vi "Autonomous Independent.vi"() -> ()   [LabVIEW 2016]
doc: "This VI is called when autonomous begins, and will automatically be terminated when autonomous ends. You can carry out timed or sensor driven robot movement independently without needing to return to the caller."
uses:
  <vilib>/Rock Robotics/WPI/Solenoid/WPI_SolenoidValue.ctl
  <vilib>/Rock Robotics/WPI/Utilities/WPI_GetSetVariantRefNum.vi
  <vilib>/Rock Robotics/Network Tables/NT Read String.vi
  <vilib>/Rock Robotics/Network Tables/NT Read Boolean.vi
  <vilib>/Rock Robotics/WPI/Solenoid/WPI_SolenoidSetEnum.vi
  <vilib>/Rock Robotics/WPI/RobotDrive/WPI_RobotDriveArcadeDrive_Standard(NoSaturation).vi
  <vilib>/Rock Robotics/Network Tables/NT Write Numeric Array.vi
  <vilib>/Rock Robotics/Network Tables/NT Write Number.vi
  Google Drive/HowdyBots-Share/BotStuff/2017_SteamWorks/Code/BotCode/Active/Robot Global Data.vi
  <vilib>/Rock Robotics/WPI/Counter/WPI_CounterDigitalInputToDigitalSource.vi
  <vilib>/Rock Robotics/SystemInterfaces/DIO/FPGA_DIOChannel.ctl
panel:
  out "Hook Center Cons":dbl
  out "gyro":dbl
  out "sonar distance (inches)":dbl
  out "Encoder Loop":dbl
  out "Encoder Loop":string
  out "Current Movement, for debugging 2":T1 {"Y Joystick Value" scale=1.0..-1.0; "X Joystick Value" scale=-1.0..1.0}
  in  "Array of robot movements 2":T2(array[cluster])=[{"X Joystick Value"=0.39393939393939403, "Y Joystick Value"=0.0, "Delay (sec)"=1.0, "Movement Name"="turn"}, {"X Joystick Value"=-0.3737373737373737, "Y Joystick Value"=0.0, "Delay (sec)"=1.0, "Movement Name"="turn back"}] {"Y Joystick Value" scale=1.0..-1.0; "X Joystick Value" scale=-1.0..1.0}
  # "Sensor Readings\nConstanly updated in\nwhile loopes"
  # "Be sure to right-click and choose Data Operations>>Make Current Value default if you want to save the array values with the VI"
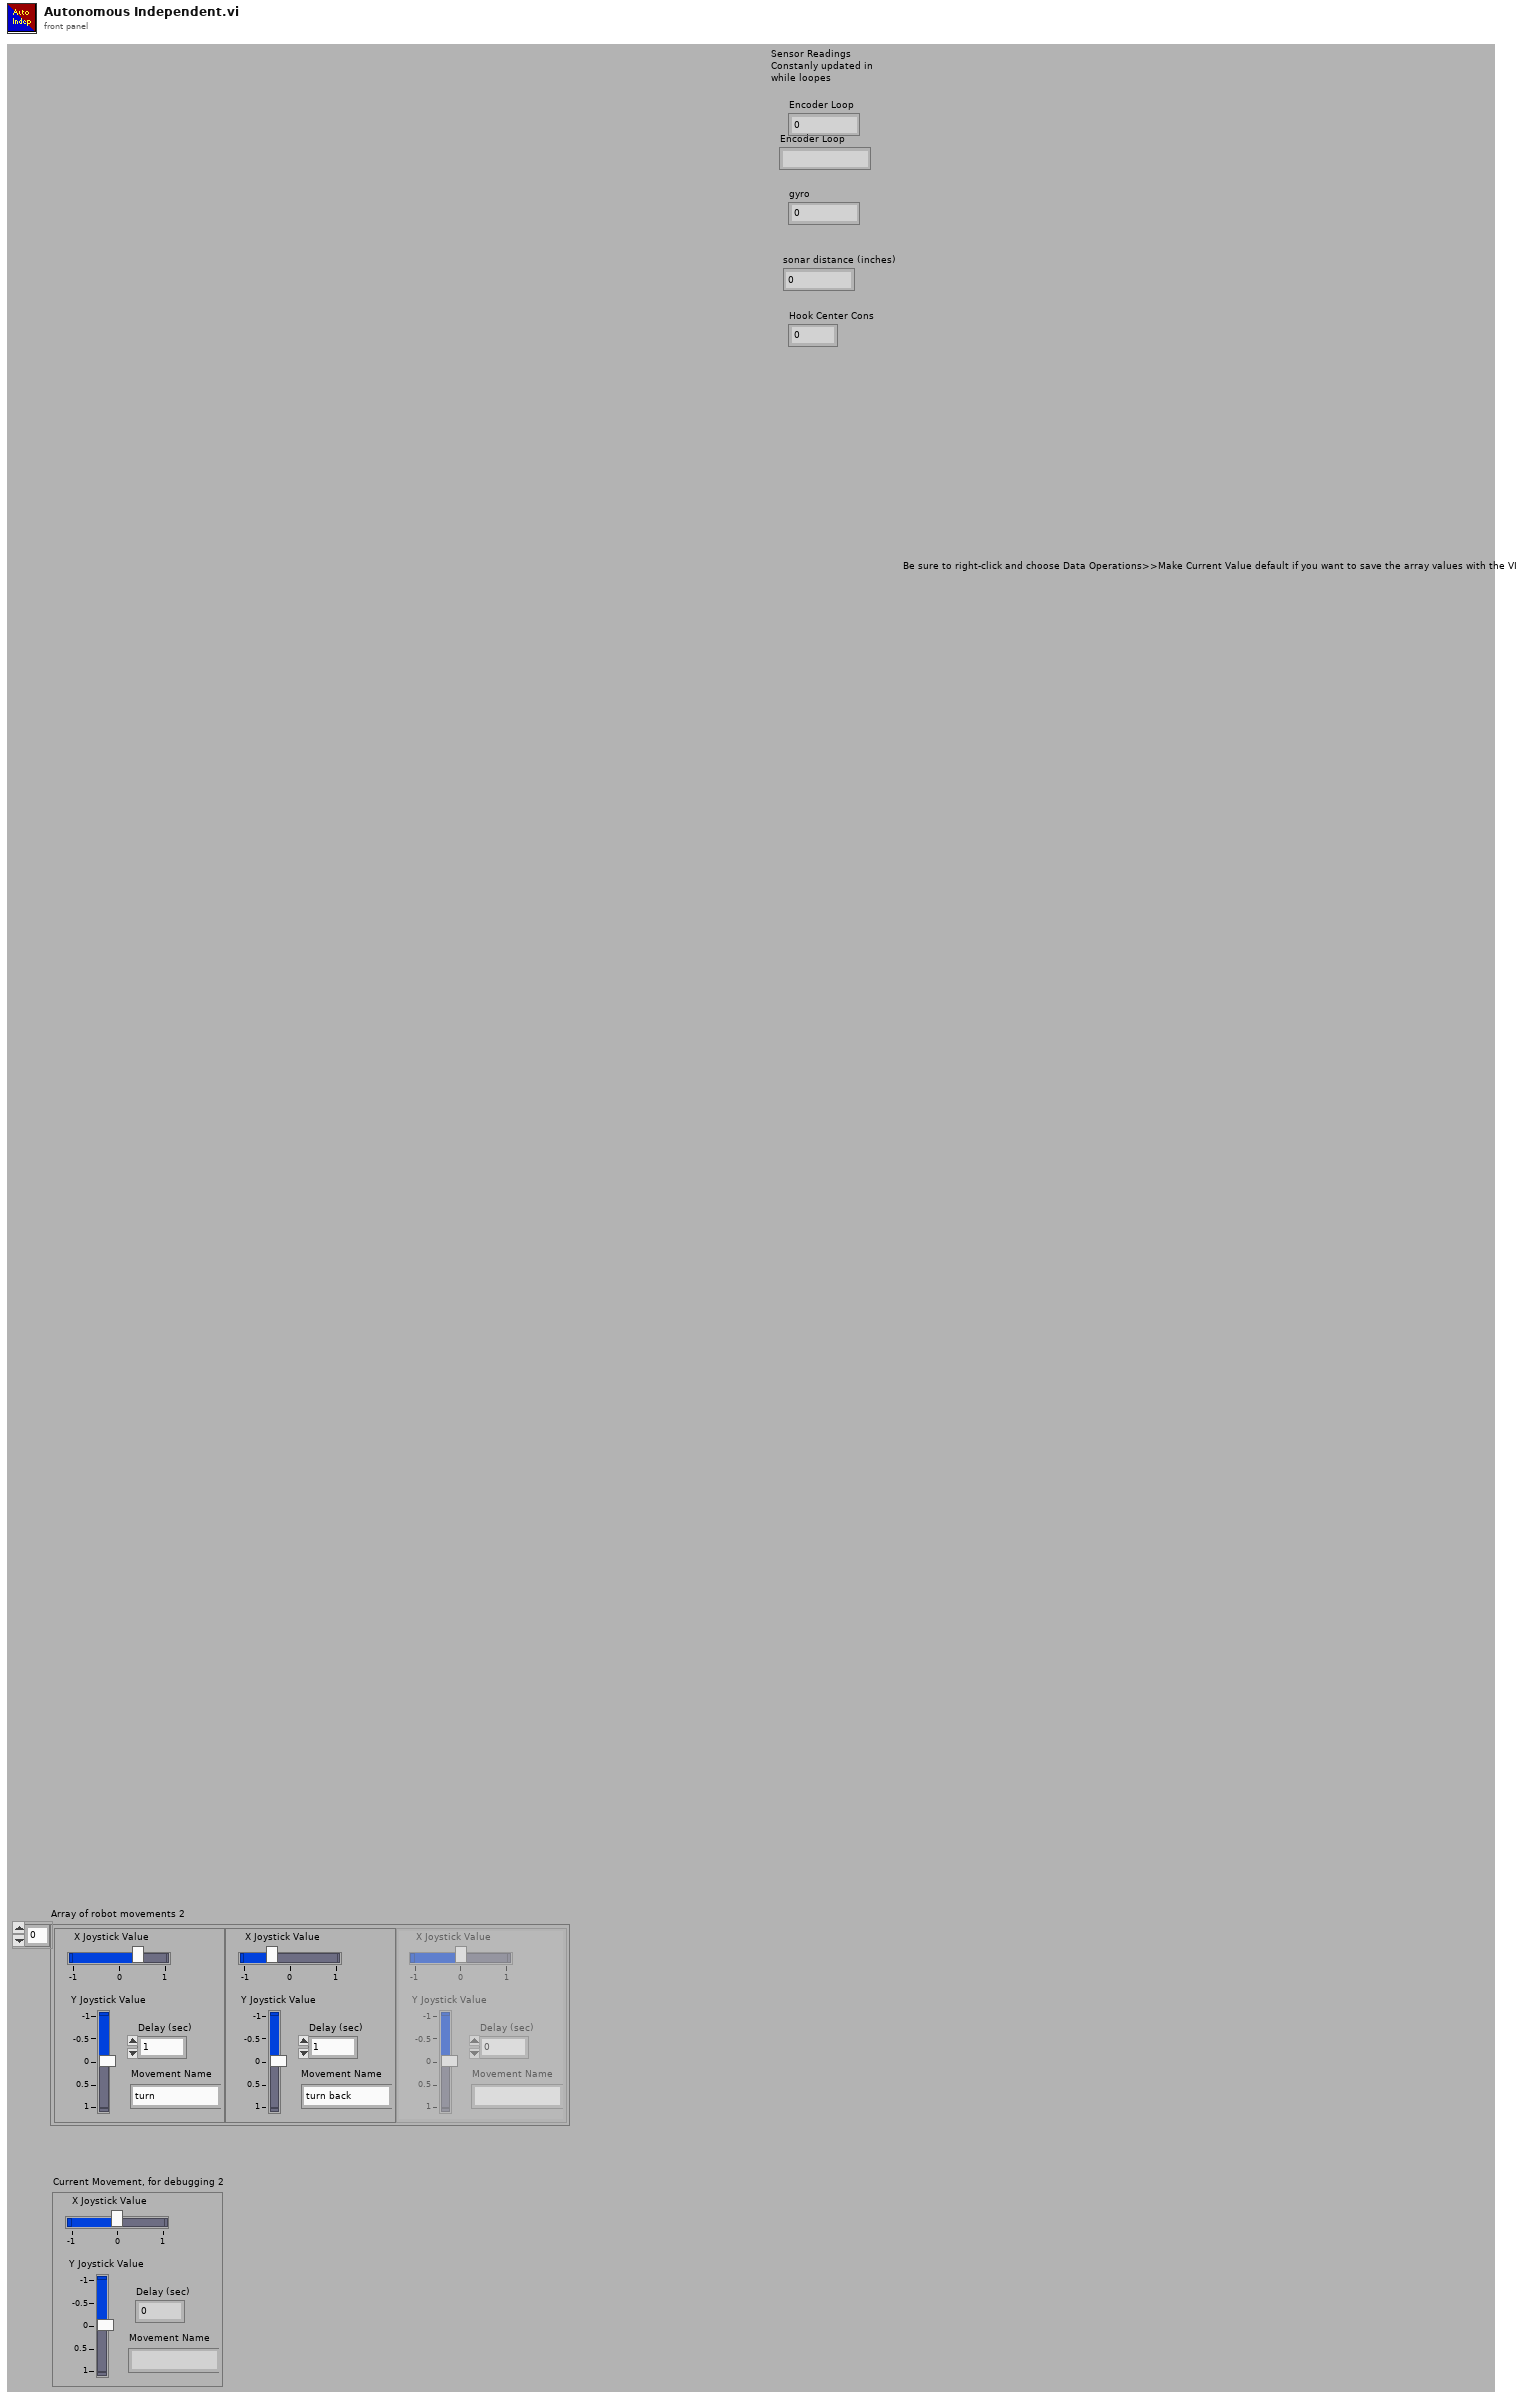
[diagram p1: front panel]
types:
  T1 = cluster{"X Joystick Value":dbl, "Y Joystick Value":dbl, "Delay (sec)":dbl, "Movement Name":string}
  T2 = cluster{"X Joystick Value":dbl, "Y Joystick Value":dbl, "Delay (sec)":dbl, "Movement Name":string}[]
  T3 = typedef "FPGA_DIOChannel.ctl" = enum8{"DIO 0", "DIO 1", "DIO 2", "DIO 3", "DIO 4", "DIO 5", "DIO 6", "DIO 7", "DIO 8", "DIO 9", "DIO MXP 0", "DIO MXP 1", "DIO MXP 2", "DIO MXP 3", "DIO MXP 4", "DIO MXP 5", "DIO MXP 6", "DIO MXP 7", "DIO MXP 8", "DIO MXP 9", "DIO MXP 10", "DIO MXP 11", "DIO MXP 12", "DIO MXP 13", "DIO MXP 14", "DIO MXP 15", "SPI Port CS1", "SPI Port CS2", "SPI Port CS3", "SPI Port MISO", "SPI Port MOSI", "Invalid"}
  T4 = typedef "WPI_DigitalInputDevRef.ctl" = cluster{"DevStatus":errorcluster, "DIO Channel":T3}
  T5 = typedef "FPGA_CounterEncoderSourceConvertionLVSourceType.ctl" = cluster{"DevStatus":errorcluster, "AnalogTriggerMode?":bool, "DigitalMode":cluster{"DIO Channel":T6}, "AnalogTriggerMode":cluster{"AnalogTriggerIndex":T7, "OutputType":T8}}
  T6 = typedef "FPGA_DIODigitalSourceChannel.ctl" = enum8{"DIO 0", "DIO 1", "DIO 2", "DIO 3", "DIO 4", "DIO 5", "DIO 6", "DIO 7", "DIO 8", "DIO 9", "DIO MXP 0", "DIO MXP 1", "DIO MXP 2", "DIO MXP 3", "DIO MXP 4", "DIO MXP 5", "DIO MXP 6", "DIO MXP 7", "DIO MXP 8", "DIO MXP 9", "DIO MXP 10", "DIO MXP 11", "DIO MXP 12", "DIO MXP 13", "DIO MXP 14", "DIO MXP 15", "Disabled"}
  T7 = typedef "FPGA_AnalogTriggerIndex.ctl" = enum8{"Trig 0", "Trig 1", "Trig 2", "Trig 3", "Trig 4", "Trig 5", "Trig 6", "Trig 7", "Invalid"}
  T8 = typedef "FPGA_AnalogTriggerOutType.ctl" = enum16{"InWindow", "TriggerState", "Rising", "Falling"}
  T9 = typedef "WPI_EncoderDevRef.ctl" = cluster{"DevStatus":errorcluster, "EncoderIndex":T10, "CounterIndex":T11, "DistancePerCount":dbl, "Decoding Type":T12}
  T10 = typedef "FPGA_EncoderIdx.ctl" = enum8{"Enc 0", "Enc 1", "Enc 2", "Enc 3", "Enc 4", "Enc 5", "Enc 6", "Enc 7", "Invalid"}
  T11 = typedef "FPGA_CounterCtrSystemIndex.ctl" = enum8{"Ctr 0", "Ctr 1", "Ctr 2", "Ctr 3", "Ctr 4", "Ctr 5", "Ctr 6", "Ctr 7", "Invalid"}
  T12 = typedef "WPI_EncoderType.ctl" = enum16{"1x", "2x", "4x"}
  T13 = typedef "WPI_JoystickDevRef.ctl" = cluster{"Device":T14}
  T14 = typedef "WPI_JoystickDeviceEnum.ctl" = enum16{"USB 0", "USB 1", "USB 2", "USB 3", "USB 4", "USB 5"}
  T15 = typedef "WPI_SolenoidValue.ctl" = enum16{"Off", "On", "Forward", "Reverse"}
  T16 = typedef "WPI_SolenoidDevRef.ctl" = cluster{"DevStatus":errorcluster, "Pneumatics Control Module":u8, "Forward Solenoid Channel":T17, "Reverse Solenoid Channel":T17}
  T17 = typedef "WPI_SolenoidChannel.ctl" = enum8{"Solenoid 0", "Solenoid 1", "Solenoid 2", "Solenoid 3", "Solenoid 4", "Solenoid 5", "Solenoid 6", "Solenoid 7", "Invalid"}
  T18 = typedef "WPI_RobotDriveDevRef.ctl" = cluster{"DevStatus":errorcluster, "Motors[]":T19[], "Square Inputs":bool, "Max Output":dbl}
  T19 = typedef "WPI_MotorControlDeviceRef.ctl" = cluster{"DeviceStatus":errorcluster, "Type":T20, "PWM":cluster{"PWM Channel":T21, "DeadBand":T22}, "CAN":cluster{"Device Number":u8, "SetOutput VI Ref":variant, "GetOutput VI Ref":variant, "Enable VI Ref":variant, "Disable VI Ref":variant, "Data":variant}, "Invert":bool}
  T20 = typedef "WPI_MotorControlType.ctl" = enum16{"PWM", "CAN"}
  T21 = typedef "FPGA_DIOPWMChannel.ctl" = enum8{"PWM 0", "PWM 1", "PWM 2", "PWM 3", "PWM 4", "PWM 5", "PWM 6", "PWM 7", "PWM 8", "PWM 9", "PWM MXP 0", "PWM MXP 1", "PWM MXP 2", "PWM MXP 3", "PWM MXP 4", "PWM MXP 5", "PWM MXP 6", "PWM MXP 7", "PWM MXP 8", "PWM MXP 9", "Invalid"}
  T22 = typedef "WPI_PWMDeadband.ctl" = cluster{"Name":string, "maxPositivePwm":i32, "minPositivePwm":i32, "centerPwm":i32, "maxNegativePwm":i32, "minNegativePwm":i32, "angularRange":u16}
  T23 = typedef "WPI_DriverStationPositionInfo.ctl" = enum16{"1", "2", "3"}
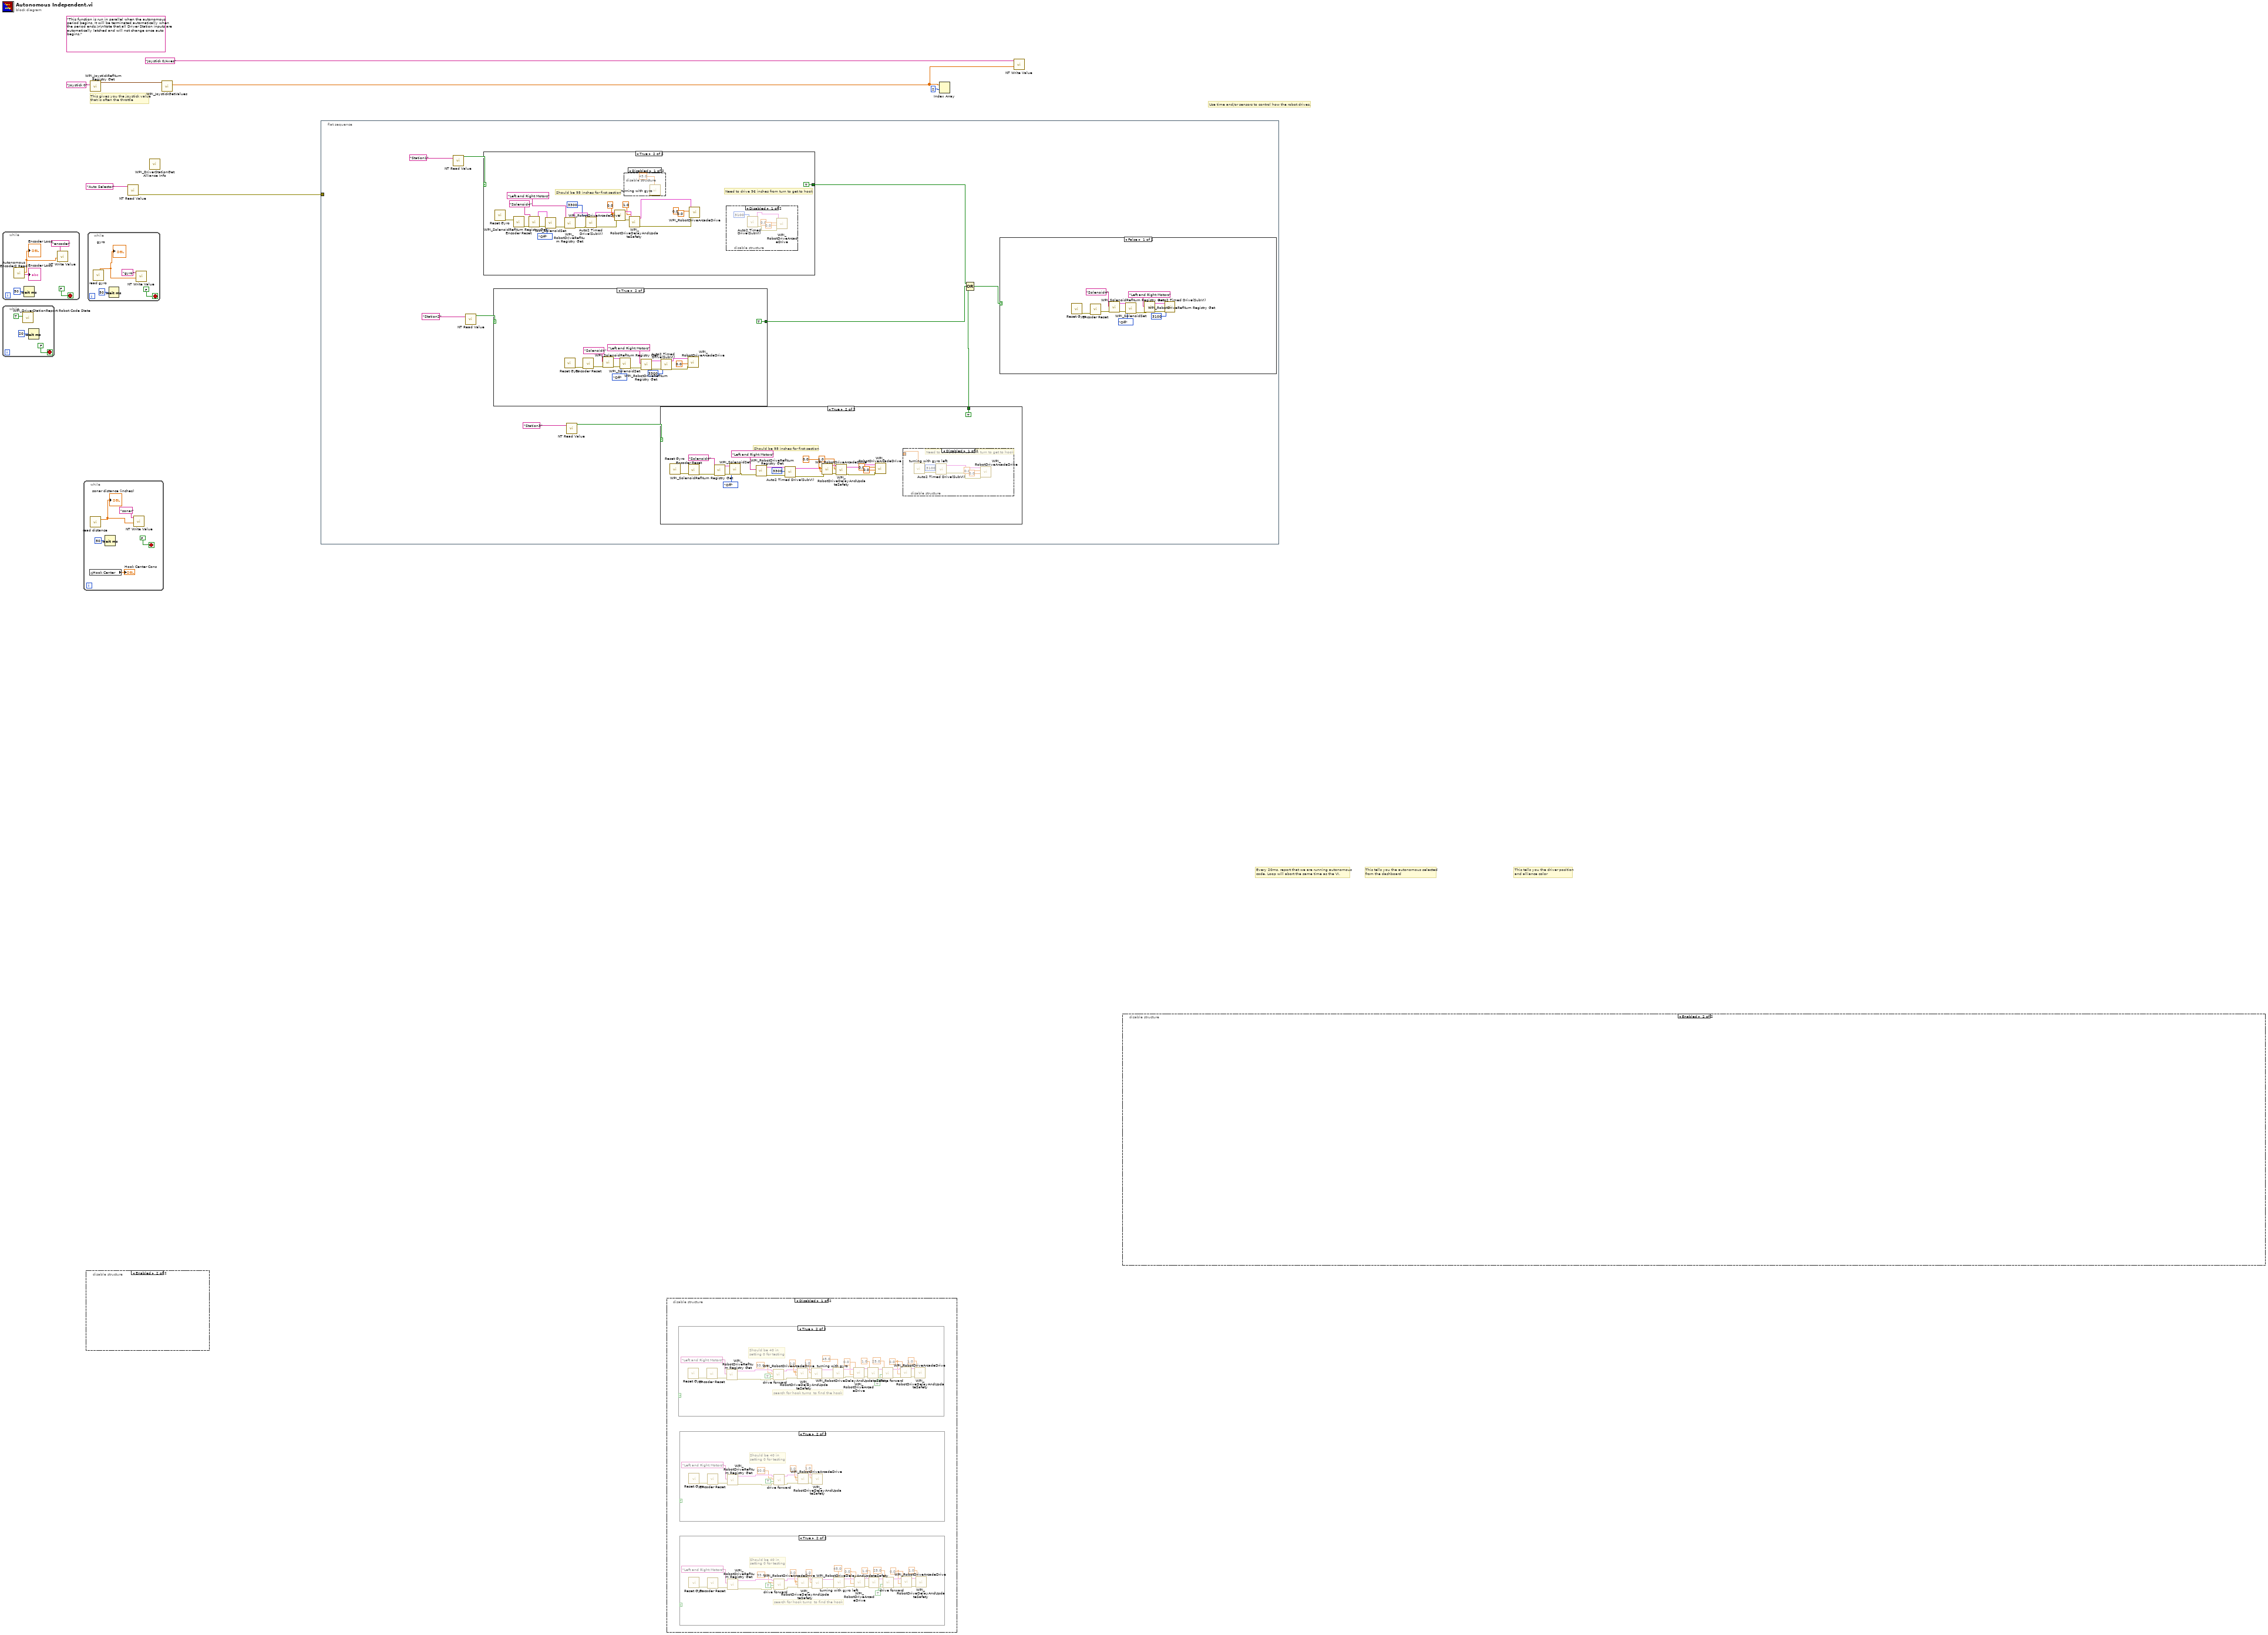
[diagram p0: block diagram]
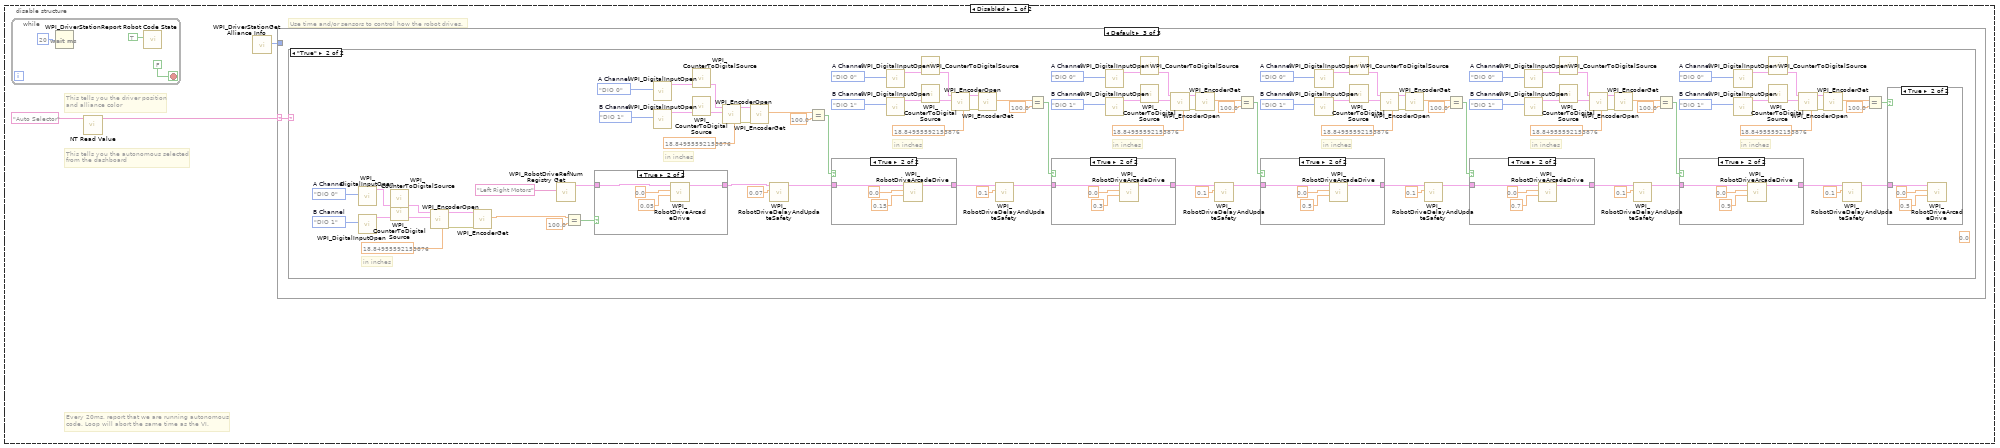
[diagram p13: hidden frame]
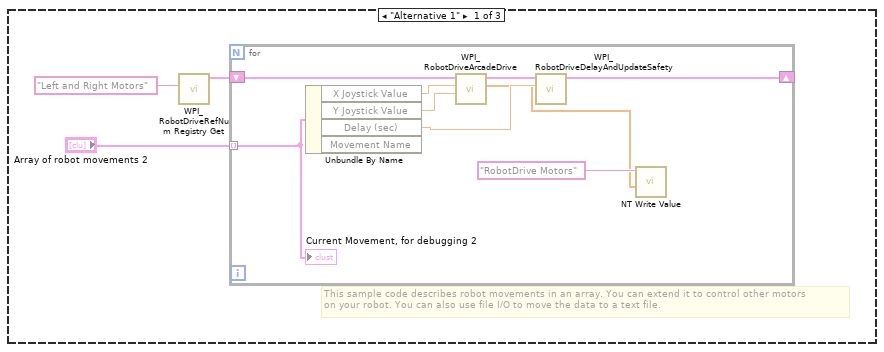
[diagram p14: hidden frame]
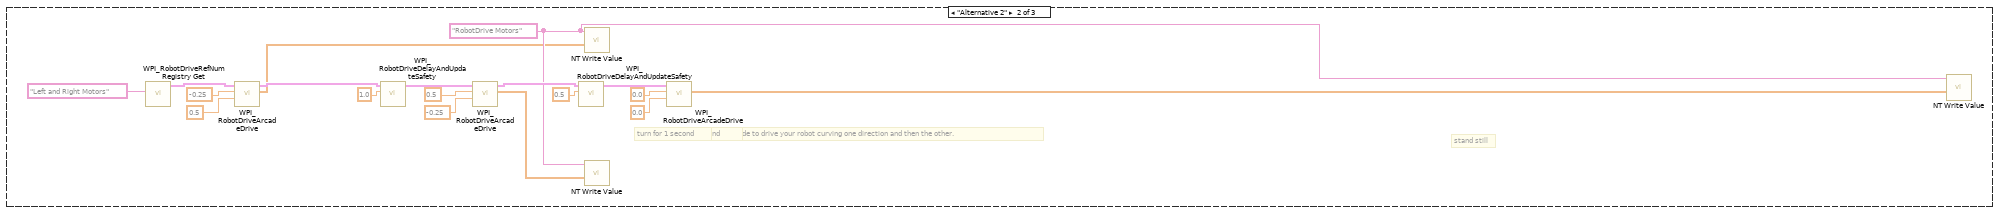
[diagram p15: hidden frame]
diagram:
  (unwired) "This function is run in parallel when the autonomous period begins. It will be terminated automatically when the period ends.\n\nNote that all Driver Station inputs are automatically latched and will not change once auto begins."
  # "This tells you the autonomous selected\nfrom the dashboard"
  # "Every 20ms, report that we are running autonomous\ncode. Loop will abort the same time as the VI."
  # "This gives you the joystick value\nthat is often the throttle"
  # "Use time and/or sensors to control how the robot drives."
  # "This tells you the driver position\nand alliance color"
  n1 = while {
    stop <- FALSE stop-if-true
    n2 = call "Autonomous Encoder2 Read.vi"() -> ("Encoder Direction"=→"Encoder Loop":string, "Encoder Distance"=w9:dbl)  [unwired: 9 in, 1 out]
    "Encoder Loop" <- w9
    n3 = Wait (ms)(milliseconds to wait=u32 50) -> ()  [unwired: 1 out]
    n4 = call-poly <vilib>:"NT Write Value.vi"("Numeric"=w9, "Name"="encoder") -> ()  [unwired: 9 in, 1 out]
  }
  n5 = while {
    stop <- FALSE stop-if-true
    n6 = call <vilib>:"WPI_DriverStationReport Robot Code State.vi"("Autonomous"=TRUE) -> ()  [unwired: 10 in, 1 out]
    n7 = Wait (ms)(milliseconds to wait=u32 20) -> ()  [unwired: 1 out]
  }
  n8 = while {
    stop <- FALSE stop-if-true
    n9 = global read "Robot Global Data.vi" "Hook Center"() -> (→"Hook Center Cons":dbl)
    n10 = call "read distance.vi"() -> ("Distance 2"=w18:dbl)  [unwired: 10 in, 1 out]
    "sonar distance (inches)" <- w18
    n11 = Wait (ms)(milliseconds to wait=u32 50) -> ()  [unwired: 1 out]
    n12 = call-poly <vilib>:"NT Write Value.vi"("Numeric"=w18, "Name"="sonar") -> ()  [unwired: 9 in, 1 out]
  }
  n13 = disable-structure shown="Enabled" {
    frame Disabled {
      w34 = FPGA_DIOChannel."DIO 1"  # B Channel
      w33 = FPGA_DIOChannel."DIO 0"  # A Channel
      # "in inches"
      n14 = call <vilib>:"WPI_DigitalInputOpen.vi"("DIO Channel"=w33) -> ("DigitalInputDevRef"=w30:T4)  [unwired: 1 in, 9 out]
      n15 = call <vilib>:"WPI_DigitalInputOpen.vi"("DIO Channel"=w34) -> ("DigitalInputDevRef"=w31:T4)  [unwired: 1 in, 9 out]
      n16 = call-poly <vilib>:"WPI_CounterToDigitalSource.vi"("DigitalInputDevRef"=w30) -> ("Digital Source"=w29:T5)  [unwired: 6 out]
      n17 = call-poly <vilib>:"WPI_CounterToDigitalSource.vi"("DigitalInputDevRef"=w31) -> ("Digital Source"=w32:T5)  [unwired: 6 out]
      n18 = call <vilib>:"WPI_EncoderOpen.vi"("DistancePerCount"=18.84955592153876, "Invert Direction (False)"=FALSE, "BSource"=w32, "ASource"=w29) -> ("error out"=w27:errorcluster, "EncoderDevRef"=w28:T9)  [unwired: 4 in, 2 out]
      n19 = call-poly <vilib>:"NT Write Value.vi"("Name"="Encoder Distance") -> ()  [unwired: 10 in, 1 out]
      n20 = call <vilib>:"WPI_EncoderRefNum Registry Set.vi"("error in (no error)"=w27, "refnum name"="Encoder", "EncoderDevRef"=w28) -> ("error out"=w25:errorcluster, "EncoderDevRef"=w26:T9)  [unwired: 7 in]
      n21 = call <vilib>:"WPI_EncoderGet.vi"("error in (no error)"=w25, "EncoderDevRef"=w26) -> ()  [unwired: 4 in, 6 out]
    }
    frame Enabled {
    }
  }
  n22 = while {
    stop <- FALSE stop-if-true
    n23 = call "read gyro.vi"() -> ("Angle 2"=w36:dbl)  [unwired: 10 in, 1 out]
    "gyro" <- w36
    n24 = Wait (ms)(milliseconds to wait=u32 50) -> ()  [unwired: 1 out]
    n25 = call-poly <vilib>:"NT Write Value.vi"("Numeric"=w36, "Name"="gyro") -> ()  [unwired: 9 in, 1 out]
  }
  n26 = call <vilib>:"WPI_JoystickRefNum Registry Get.vi"("refnum name"="Joystick 0") -> ("JoystickDevRef"=w6:T13)  [unwired: 1 in, 9 out]
  n27 = call-poly <vilib>:"NT Read Value.vi"("Name"="Auto Selector") -> ("error out"=w1:errorcluster)  [unwired: 9 in, 1 out]
  n28 = call <vilib>:"WPI_DriverStationGet Alliance Info.vi"() -> ()  [unwired: 12 out]
  n29 = call <vilib>:"WPI_JoystickGetValues.vi"("JoystickDevRef"=w6) -> ("Axes"=w3:dbl[])  [unwired: 6 in, 4 out]
  n30 = flat-sequence {
    tunnel: w1 -> [_]
    frame #0 {
      n31 = call-poly <vilib>:"NT Read Value.vi"("Name"="Station1") -> ("Boolean"=w43:bool)  [unwired: 9 in, 1 out]
      n32 = call-poly <vilib>:"NT Read Value.vi"("Name"="Station2") -> ("Boolean"=w47:bool)  [unwired: 9 in, 1 out]
      n33 = case shown="True" w43 {
        selector: w43 -> [w60 _]
        tunnel: [w60 TRUE] -> w42
        frame False {
        }
        frame True {
          (unwired) 0.0 ("Y axis value")
          w76 = 0.0 ("X axis value")
          # "Need to drive 96 inches from turn to get to hook"
          # "Should be 95 inches for first section"
          n34 = call "Reset Gyro.vi"() -> ("error out"=w80:errorcluster)  [unwired: 11 in]
          n35 = call "Encoder Reset.vi"("error in (no error)"=w80) -> ("error out"=w69:errorcluster)  [unwired: 10 in]
          n36 = call <vilib>:"WPI_SolenoidRefNum Registry Get.vi"("error in (no error)"=w69, "refnum name"="Solenoid4") -> ("error out"=w68:errorcluster, "SolenoidDevRef"=w65:T16)  [unwired: 8 in]
          n37 = call-poly <vilib>:"WPI_SolenoidSet.vi"("error in (no error)"=w68, "Value"=WPI_SolenoidValue."Off", "SolenoidDevRef"=w65) -> ("error out"=w66:errorcluster)  [unwired: 7 in, 1 out]
          n38 = call <vilib>:"WPI_RobotDriveRefNum Registry Get.vi"("error in (no error)"=w66, "refnum name"="Left and Right Motors") -> ("error out"=w74:errorcluster, "RobotDriveDevRef"=w75:T18)  [unwired: 8 out]
          n39 = call "Auto2 Timed Drive(SubVI).vi"("error in (no error)"=w74, "milliseconds to wait"=u32 3300, "RobotDriveDevRef in"=w75) -> ("error out"=w72:errorcluster, "RobotDriveDevRef out"=w73:T18)  [unwired: 7 in]
          n40 = call-poly <vilib>:"WPI_RobotDriveArcadeDrive.vi"("error in (no error)"=w72, "Y axis value"=w76, "X axis value"=w76, "RobotDriveDevRef"=w73) -> ("error out"=w78:errorcluster, "RobotDriveDevRef"=w79:T18)  [unwired: 6 out]
          n41 = disable-structure shown="Disabled" {
            frame Disabled {
              n42 = call "turning with gyro.vi"("desired angle"=45.0) -> ("RobotDriveDevRef"=w83:T18)  [unwired: 8 in, 2 out]
            }
            frame Enabled {
            }
          }
          n43 = call <vilib>:"WPI_RobotDriveDelayAndUpdateSafety.vi"("error in (no error)"=w78, "Delay (s)"=1.0, "RobotDriveDevRef"=w79) -> ("error out"=w61:errorcluster, "RobotDriveDevRef 2"=w62:T18)  [unwired: 7 in]
          n44 = call-poly <vilib>:"WPI_RobotDriveArcadeDrive.vi"("error in (no error)"=w61, "X axis value"=0.0, "RobotDriveDevRef"=w62) -> ()  [unwired: 6 in, 3 out]
          n45 = disable-structure shown="Disabled" {
            frame Disabled {
              n46 = call "Auto2 Timed Drive(SubVI).vi"("milliseconds to wait"=u32 3100) -> ("error out"=w85:errorcluster, "RobotDriveDevRef out"=w86:T18)  [unwired: 9 in]
              n47 = call-poly <vilib>:"WPI_RobotDriveArcadeDrive.vi"("error in (no error)"=w85, "Y axis value"=0.0, "X axis value"=0.0, "RobotDriveDevRef"=w86) -> ()  [unwired: 5 in, 3 out]
            }
            frame Enabled {
            }
          }
        }
      }
      n48 = case shown="True" w47 {
        selector: w47 -> [w120 _]
        tunnel: [w120 TRUE] -> w41
        frame False {
        }
        frame True {
          n49 = call "Reset Gyro.vi"() -> ("error out"=w134:errorcluster)  [unwired: 11 in]
          n50 = call "Encoder Reset.vi"("error in (no error)"=w134) -> ("error out"=w125:errorcluster)  [unwired: 10 in]
          n51 = call <vilib>:"WPI_SolenoidRefNum Registry Get.vi"("error in (no error)"=w125, "refnum name"="Solenoid4") -> ("error out"=w129:errorcluster, "SolenoidDevRef"=w127:T16)  [unwired: 8 in]
          n52 = call-poly <vilib>:"WPI_SolenoidSet.vi"("error in (no error)"=w129, "Value"=WPI_SolenoidValue."Off", "SolenoidDevRef"=w127) -> ("error out"=w124:errorcluster)  [unwired: 7 in, 1 out]
          n53 = call <vilib>:"WPI_RobotDriveRefNum Registry Get.vi"("error in (no error)"=w124, "refnum name"="Left and Right Motors") -> ("error out"=w132:errorcluster, "RobotDriveDevRef"=w133:T18)  [unwired: 8 out]
          n54 = call "Auto2 Timed Drive(SubVI).vi"("error in (no error)"=w132, "milliseconds to wait"=u32 3300, "RobotDriveDevRef in"=w133) -> ("error out"=w121:errorcluster, "RobotDriveDevRef out"=w123:T18)  [unwired: 7 in]
          n55 = call-poly <vilib>:"WPI_RobotDriveArcadeDrive.vi"("error in (no error)"=w121, "Y axis value"=0.0, "RobotDriveDevRef"=w123) -> ()  [unwired: 6 in, 3 out]
        }
      }
      n56 = call-poly <vilib>:"NT Read Value.vi"("Name"="Station3") -> ("Boolean"=w45:bool)  [unwired: 9 in, 1 out]
      n57 = case shown="True" w45 {
        selector: w45 -> [w89 _]
        tunnel: [w89 TRUE] -> w40
        frame False {
        }
        frame True {
          w106 = 0.0 ("X axis value")
          # "Should be 95 inches for first section"
          n58 = call "Reset Gyro.vi"() -> ("error out"=w110:errorcluster)  [unwired: 11 in]
          n59 = call "Encoder Reset.vi"("error in (no error)"=w110) -> ("error out"=w96:errorcluster)  [unwired: 10 in]
          n60 = call <vilib>:"WPI_SolenoidRefNum Registry Get.vi"("error in (no error)"=w96, "refnum name"="Solenoid4") -> ("error out"=w99:errorcluster, "SolenoidDevRef"=w97:T16)  [unwired: 8 in]
          n61 = call-poly <vilib>:"WPI_SolenoidSet.vi"("error in (no error)"=w99, "Value"=WPI_SolenoidValue."Off", "SolenoidDevRef"=w97) -> ("error out"=w95:errorcluster)  [unwired: 7 in, 1 out]
          n62 = call <vilib>:"WPI_RobotDriveRefNum Registry Get.vi"("error in (no error)"=w95, "refnum name"="Left and Right Motors") -> ("error out"=w104:errorcluster, "RobotDriveDevRef"=w105:T18)  [unwired: 8 out]
          n63 = call "Auto2 Timed Drive(SubVI).vi"("error in (no error)"=w104, "milliseconds to wait"=u32 3300, "RobotDriveDevRef in"=w105) -> ("error out"=w102:errorcluster, "RobotDriveDevRef out"=w103:T18)  [unwired: 7 in]
          n64 = call-poly <vilib>:"WPI_RobotDriveArcadeDrive.vi"("error in (no error)"=w102, "Y axis value"=w106, "X axis value"=w106, "RobotDriveDevRef"=w103) -> ("error out"=w108:errorcluster, "RobotDriveDevRef"=w109:T18)  [unwired: 6 out]
          n65 = call <vilib>:"WPI_RobotDriveDelayAndUpdateSafety.vi"("error in (no error)"=w108, "Delay (s)"=1.0, "RobotDriveDevRef"=w109) -> ("error out"=w91:errorcluster, "RobotDriveDevRef 2"=w90:T18)  [unwired: 7 in]
          n66 = call-poly <vilib>:"WPI_RobotDriveArcadeDrive.vi"("error in (no error)"=w91, "Y axis value"=0.0, "X axis value"=0.0, "RobotDriveDevRef"=w90) -> ()  [unwired: 5 in, 3 out]
          n67 = disable-structure shown="Disabled" {
            disable-tunnel: _ -> [w119 _]
            frame Disabled {
              # "Need to drive 96 inches from turn to get to hook"
              n68 = call "turning with gyro left.vi"("desired angle"=w119) -> ("error out"=w117:errorcluster, "RobotDriveDevRef 2"=w118:T18)  [unwired: 8 in, 1 out]
              n69 = call "Auto2 Timed Drive(SubVI).vi"("error in (no error)"=w117, "milliseconds to wait"=u32 3100, "RobotDriveDevRef in"=w118) -> ("error out"=w113:errorcluster, "RobotDriveDevRef out"=w114:T18)  [unwired: 7 in]
              n70 = call-poly <vilib>:"WPI_RobotDriveArcadeDrive.vi"("error in (no error)"=w113, "Y axis value"=0.0, "X axis value"=0.0, "RobotDriveDevRef"=w114) -> ()  [unwired: 5 in, 3 out]
            }
            frame Enabled {
            }
          }
        }
      }
      n71 = Compound Arithmetic op=OR(w42, w41, w40) -> (w39:bool)
      n72 = case shown="False" w39 {
        frame False {
          n73 = call "Reset Gyro.vi"() -> ("error out"=w58:errorcluster)  [unwired: 11 in]
          n74 = call "Encoder Reset.vi"("error in (no error)"=w58) -> ("error out"=w50:errorcluster)  [unwired: 10 in]
          n75 = call <vilib>:"WPI_SolenoidRefNum Registry Get.vi"("error in (no error)"=w50, "refnum name"="Solenoid4") -> ("error out"=w54:errorcluster, "SolenoidDevRef"=w52:T16)  [unwired: 8 in]
          n76 = call-poly <vilib>:"WPI_SolenoidSet.vi"("error in (no error)"=w54, "Value"=WPI_SolenoidValue."Off", "SolenoidDevRef"=w52) -> ("error out"=w49:errorcluster)  [unwired: 7 in, 1 out]
          n77 = call <vilib>:"WPI_RobotDriveRefNum Registry Get.vi"("error in (no error)"=w49, "refnum name"="Left and Right Motors") -> ("error out"=w56:errorcluster, "RobotDriveDevRef"=w57:T18)  [unwired: 8 out]
          n78 = call "Auto2 Timed Drive(SubVI).vi"("error in (no error)"=w56, "milliseconds to wait"=u32 3100, "RobotDriveDevRef in"=w57) -> ()  [unwired: 7 in, 2 out]
        }
        frame True {
        }
      }
    }
  }
  n79 = disable-structure shown="Disabled" {
    frame Disabled {
      n80 = case shown="True" {
        selector: _ -> [_ _]
        frame False {
        }
        frame True {
          w184 = 0.0 ("X axis value")
          w195 = 0.0 ("X axis value")
          w202 = 0.0 ("X axis value")
          # "search for hook turns  to find the hook"
          # "Should be 40 in\nsetting 0 for testing"
          n81 = call "Reset Gyro.vi"() -> ("error out"=w209:errorcluster)  [unwired: 11 in]
          n82 = call "Encoder Reset.vi"("error in (no error)"=w209) -> ("error out"=w211:errorcluster)  [unwired: 10 in]
          n83 = call <vilib>:"WPI_RobotDriveRefNum Registry Get.vi"("error in (no error)"=w211, "refnum name"="Left and Right Motors") -> ("error out"=w208:errorcluster, "RobotDriveDevRef"=w210:T18)  [unwired: 8 out]
          n84 = call "drive forward.vi"("error in (no error)"=w208, "forward"=TRUE, "desired distance"=95.0, "RobotDriveDevRef in"=w210) -> ("error out"=w200:errorcluster, "RobotDriveDevRef out"=w201:T18)  [unwired: 6 in]
          n85 = call-poly <vilib>:"WPI_RobotDriveArcadeDrive.vi"("error in (no error)"=w200, "Y axis value"=w202, "X axis value"=w202, "RobotDriveDevRef"=w201) -> ("error out"=w204:errorcluster, "RobotDriveDevRef"=w205:T18)  [unwired: 6 out]
          n86 = call <vilib>:"WPI_RobotDriveDelayAndUpdateSafety.vi"("error in (no error)"=w204, "Delay (s)"=1.0, "RobotDriveDevRef"=w205) -> ("error out"=w198:errorcluster, "RobotDriveDevRef 2"=w199:T18)  [unwired: 7 in]
          n87 = call "turning with gyro.vi"("desired angle"=45.0, "error in (no error)"=w198, "RobotDriveDevRef"=w199) -> ("error out"=w192:errorcluster, "RobotDriveDevRef 2"=w196:T18)  [unwired: 7 in]
          n88 = call-poly <vilib>:"WPI_RobotDriveArcadeDrive.vi"("error in (no error)"=w192, "Y axis value"=w195, "X axis value"=w195, "RobotDriveDevRef"=w196) -> ("error out"=w193:errorcluster, "RobotDriveDevRef"=w194:T18)  [unwired: 6 out]
          n89 = call <vilib>:"WPI_RobotDriveDelayAndUpdateSafety.vi"("error in (no error)"=w193, "Delay (s)"=1.0, "RobotDriveDevRef"=w194) -> ("error out"=w190:errorcluster, "RobotDriveDevRef 2"=w189:T18)  [unwired: 7 in]
          n90 = call "drive forward.vi"("error in (no error)"=w190, "forward"=TRUE, "desired distance"=25.0, "RobotDriveDevRef in"=w189) -> ("error out"=w185:errorcluster, "RobotDriveDevRef out"=w186:T18)  [unwired: 6 in]
          n91 = call-poly <vilib>:"WPI_RobotDriveArcadeDrive.vi"("error in (no error)"=w185, "Y axis value"=w184, "X axis value"=w184, "RobotDriveDevRef"=w186) -> ("error out"=w182:errorcluster, "RobotDriveDevRef"=w183:T18)  [unwired: 6 out]
          n92 = call <vilib>:"WPI_RobotDriveDelayAndUpdateSafety.vi"("error in (no error)"=w182, "Delay (s)"=1.0, "RobotDriveDevRef"=w183) -> ()  [unwired: 7 in, 2 out]
        }
      }
      n93 = case shown="True" {
        selector: _ -> [_ _]
        frame False {
        }
        frame True {
          w170 = 0.0 ("X axis value")
          # "Should be 40 in\nsetting 0 for testing"
          n94 = call "Reset Gyro.vi"() -> ("error out"=w177:errorcluster)  [unwired: 11 in]
          n95 = call "Encoder Reset.vi"("error in (no error)"=w177) -> ("error out"=w179:errorcluster)  [unwired: 10 in]
          n96 = call <vilib>:"WPI_RobotDriveRefNum Registry Get.vi"("error in (no error)"=w179, "refnum name"="Left and Right Motors") -> ("error out"=w176:errorcluster, "RobotDriveDevRef"=w178:T18)  [unwired: 8 out]
          n97 = call "drive forward.vi"("error in (no error)"=w176, "forward"=TRUE, "desired distance"=60.0, "RobotDriveDevRef in"=w178) -> ("error out"=w168:errorcluster, "RobotDriveDevRef out"=w169:T18)  [unwired: 6 in]
          n98 = call-poly <vilib>:"WPI_RobotDriveArcadeDrive.vi"("error in (no error)"=w168, "Y axis value"=w170, "X axis value"=w170, "RobotDriveDevRef"=w169) -> ("error out"=w172:errorcluster, "RobotDriveDevRef"=w173:T18)  [unwired: 6 out]
          n99 = call <vilib>:"WPI_RobotDriveDelayAndUpdateSafety.vi"("error in (no error)"=w172, "Delay (s)"=1.0, "RobotDriveDevRef"=w173) -> ()  [unwired: 7 in, 2 out]
        }
      }
      n100 = case shown="True" {
        selector: _ -> [_ _]
        frame False {
        }
        frame True {
          w139 = 0.0 ("X axis value")
          w150 = 0.0 ("X axis value")
          w157 = 0.0 ("X axis value")
          # "search for hook turns  to find the hook"
          # "Should be 40 in\nsetting 0 for testing"
          n101 = call "Reset Gyro.vi"() -> ("error out"=w164:errorcluster)  [unwired: 11 in]
          n102 = call "Encoder Reset.vi"("error in (no error)"=w164) -> ("error out"=w166:errorcluster)  [unwired: 10 in]
          n103 = call <vilib>:"WPI_RobotDriveRefNum Registry Get.vi"("error in (no error)"=w166, "refnum name"="Left and Right Motors") -> ("error out"=w163:errorcluster, "RobotDriveDevRef"=w165:T18)  [unwired: 8 out]
          n104 = call "drive forward.vi"("error in (no error)"=w163, "forward"=TRUE, "desired distance"=95.0, "RobotDriveDevRef in"=w165) -> ("error out"=w155:errorcluster, "RobotDriveDevRef out"=w156:T18)  [unwired: 6 in]
          n105 = call-poly <vilib>:"WPI_RobotDriveArcadeDrive.vi"("error in (no error)"=w155, "Y axis value"=w157, "X axis value"=w157, "RobotDriveDevRef"=w156) -> ("error out"=w159:errorcluster, "RobotDriveDevRef"=w160:T18)  [unwired: 6 out]
          n106 = call <vilib>:"WPI_RobotDriveDelayAndUpdateSafety.vi"("error in (no error)"=w159, "Delay (s)"=1.0, "RobotDriveDevRef"=w160) -> ("error out"=w153:errorcluster, "RobotDriveDevRef 2"=w154:T18)  [unwired: 7 in]
          n107 = call "turning with gyro left.vi"("desired angle"=45.0, "error in (no error)"=w153, "RobotDriveDevRef"=w154) -> ("error out"=w147:errorcluster, "RobotDriveDevRef 2"=w151:T18)  [unwired: 6 in, 1 out]
          n108 = call-poly <vilib>:"WPI_RobotDriveArcadeDrive.vi"("error in (no error)"=w147, "Y axis value"=w150, "X axis value"=w150, "RobotDriveDevRef"=w151) -> ("error out"=w148:errorcluster, "RobotDriveDevRef"=w149:T18)  [unwired: 6 out]
          n109 = call <vilib>:"WPI_RobotDriveDelayAndUpdateSafety.vi"("error in (no error)"=w148, "Delay (s)"=1.0, "RobotDriveDevRef"=w149) -> ("error out"=w145:errorcluster, "RobotDriveDevRef 2"=w144:T18)  [unwired: 7 in]
          n110 = call "drive forward.vi"("error in (no error)"=w145, "forward"=TRUE, "desired distance"=25.0, "RobotDriveDevRef in"=w144) -> ("error out"=w140:errorcluster, "RobotDriveDevRef out"=w141:T18)  [unwired: 6 in]
          n111 = call-poly <vilib>:"WPI_RobotDriveArcadeDrive.vi"("error in (no error)"=w140, "Y axis value"=w139, "X axis value"=w139, "RobotDriveDevRef"=w141) -> ("error out"=w137:errorcluster, "RobotDriveDevRef"=w138:T18)  [unwired: 6 out]
          n112 = call <vilib>:"WPI_RobotDriveDelayAndUpdateSafety.vi"("error in (no error)"=w137, "Delay (s)"=1.0, "RobotDriveDevRef"=w138) -> ()  [unwired: 7 in, 2 out]
        }
      }
    }
    frame Enabled {
    }
  }
  n113 = Index Array(array=w3, index #1=2 ("index")) -> ()  [unwired: 1 in, 2 out]
  n114 = call-poly <vilib>:"NT Write Value.vi"("Numeric Array"=w3, "Name"="Joystick 0/Axes") -> ()  [unwired: 9 in, 1 out]
  n115 = disable-structure shown="Enabled" {
    frame Disabled {
      # "This tells you the autonomous selected\nfrom the dashboard"
      # "Every 20ms, report that we are running autonomous\ncode. Loop will abort the same time as the VI."
      # "Use time and/or sensors to control how the robot drives."
      # "This tells you the driver position\nand alliance color"
      n116 = while {
        stop <- FALSE stop-if-true
        n117 = Wait (ms)(milliseconds to wait=u32 20) -> ()  [unwired: 1 out]
        n118 = call <vilib>:"WPI_DriverStationReport Robot Code State.vi"("Autonomous"=TRUE) -> ()  [unwired: 10 in, 1 out]
      }
      n119 = call-poly <vilib>:"NT Read Value.vi"("Name"="Auto Selector") -> ("String"=w215:string)  [unwired: 9 in, 1 out]
      n120 = call <vilib>:"WPI_DriverStationGet Alliance Info.vi"() -> ("Position"=w214:T23)  [unwired: 11 out]
      n121 = case shown="Default" w215 {
        selector: w215 -> [_ _ w246]
        tunnel: w214 -> [_ _ _]
        frame "Alternative 1" {
          # "This sample code describes robot movements in an array. You can extend it to control other motors\non your robot. You can also use file I/O to move the data to a text file."
          n122 = call <vilib>:"WPI_RobotDriveRefNum Registry Get.vi"("refnum name"="Left and Right Motors") -> ("RobotDriveDevRef"=w217:T18)  [unwired: 1 in, 9 out]
          n123 = for {
            shift-right: [w225] -> _
            shift-left: w217 -> [w226]
            tunnel: "Array of robot movements 2" -> [w221] mode=indexing
            n124 = Unbundle By Name(w221) -> ("X Joystick Value"=w224:dbl, "Y Joystick Value"=w223:dbl, "Delay (sec)"=w222:dbl)  [unwired: 1 out]
            n125 = call-poly <vilib>:"WPI_RobotDriveArcadeDrive.vi"("Y axis value"=w223, "X axis value"=w224, "RobotDriveDevRef"=w226) -> ("Motor Values"=w219:dbl[], "RobotDriveDevRef"=w227:T18)  [unwired: 1 in, 6 out]
            n126 = call <vilib>:"WPI_RobotDriveDelayAndUpdateSafety.vi"("Delay (s)"=w222, "RobotDriveDevRef"=w227) -> ("RobotDriveDevRef 2"=w225:T18)  [unwired: 8 in, 1 out]
            n127 = call-poly <vilib>:"NT Write Value.vi"("Numeric Array"=w219, "Name"="RobotDrive Motors") -> ()  [unwired: 9 in, 1 out]
            "Current Movement, for debugging 2" <- w221
          }
        }
        frame "Alternative 2" {
          w229 = "RobotDrive Motors" ("Name")
          # "This is some simple sample code to drive your robot curving one direction and then the other."
          # "stand still"
          # "other way for 0.5 second"
          # "turn for 1 second"
          n128 = call <vilib>:"WPI_RobotDriveRefNum Registry Get.vi"("refnum name"="Left and Right Motors") -> ("RobotDriveDevRef"=w245:T18)  [unwired: 1 in, 9 out]
          n129 = call-poly <vilib>:"WPI_RobotDriveArcadeDrive.vi"("Y axis value"=0.5 ("X axis value"), "X axis value"=-0.25, "RobotDriveDevRef"=w245) -> ("Motor Values"=w228:dbl[], "RobotDriveDevRef"=w238:T18)  [unwired: 1 in, 6 out]
          n130 = call <vilib>:"WPI_RobotDriveDelayAndUpdateSafety.vi"("Delay (s)"=1.0, "RobotDriveDevRef"=w238) -> ("RobotDriveDevRef 2"=w239:T18)  [unwired: 8 in, 1 out]
          n131 = call-poly <vilib>:"WPI_RobotDriveArcadeDrive.vi"("Y axis value"=-0.25 ("X axis value"), "X axis value"=0.5, "RobotDriveDevRef"=w239) -> ("Motor Values"=w230:dbl[], "RobotDriveDevRef"=w240:T18)  [unwired: 1 in, 6 out]
          n132 = call <vilib>:"WPI_RobotDriveDelayAndUpdateSafety.vi"("Delay (s)"=0.5, "RobotDriveDevRef"=w240) -> ("RobotDriveDevRef 2"=w241:T18)  [unwired: 8 in, 1 out]
          n133 = call-poly <vilib>:"NT Write Value.vi"("Numeric Array"=w228, "Name"=w229) -> ()  [unwired: 9 in, 1 out]
          n134 = call-poly <vilib>:"NT Write Value.vi"("Numeric Array"=w230, "Name"=w229) -> ()  [unwired: 9 in, 1 out]
          n135 = call-poly <vilib>:"WPI_RobotDriveArcadeDrive.vi"("Y axis value"=0.0 ("X axis value"), "X axis value"=0.0, "RobotDriveDevRef"=w241) -> ("Motor Values"=w231:dbl[])  [unwired: 1 in, 7 out]
          n136 = call-poly <vilib>:"NT Write Value.vi"("Numeric Array"=w231, "Name"=w229) -> ()  [unwired: 9 in, 1 out]
        }
        frame Default {
          n137 = case shown="\"True\"" w246 {
            frame "False", Default {
            }
            frame "True" {
              w259 = FPGA_DIOChannel."DIO 1"  # B Channel
              w258 = FPGA_DIOChannel."DIO 0"  # A Channel
              w272 = FPGA_DIOChannel."DIO 1"  # B Channel
              w271 = FPGA_DIOChannel."DIO 0"  # A Channel
              w283 = FPGA_DIOChannel."DIO 1"  # B Channel
              w282 = FPGA_DIOChannel."DIO 0"  # A Channel
              w295 = FPGA_DIOChannel."DIO 1"  # B Channel
              w294 = FPGA_DIOChannel."DIO 0"  # A Channel
              w307 = FPGA_DIOChannel."DIO 1"  # B Channel
              w306 = FPGA_DIOChannel."DIO 0"  # A Channel
              w319 = FPGA_DIOChannel."DIO 1"  # B Channel
              w318 = FPGA_DIOChannel."DIO 0"  # A Channel
              w330 = FPGA_DIOChannel."DIO 1"  # B Channel
              w329 = FPGA_DIOChannel."DIO 0"  # A Channel
              (unwired) 0.0 ("Distance")
              # "in inches"
              # "in inches"
              # "in inches"
              # "in inches"
              # "in inches"
              # "in inches"
              # "in inches"
              n138 = call <vilib>:"WPI_DigitalInputOpen.vi"("DIO Channel"=w329) -> ("DigitalInputDevRef"=w326:T4)  [unwired: 1 in, 9 out]
              n139 = call <vilib>:"WPI_DigitalInputOpen.vi"("DIO Channel"=w330) -> ("DigitalInputDevRef"=w327:T4)  [unwired: 1 in, 9 out]
              n140 = call-poly <vilib>:"WPI_CounterToDigitalSource.vi"("DigitalInputDevRef"=w326) -> ("Digital Source"=w247:T5)  [unwired: 6 out]
              n141 = call-poly <vilib>:"WPI_CounterToDigitalSource.vi"("DigitalInputDevRef"=w327) -> ("Digital Source"=w328:T5)  [unwired: 6 out]
              n142 = call <vilib>:"WPI_EncoderOpen.vi"("DistancePerCount"=18.84955592153876, "BSource"=w328, "ASource"=w247) -> ("error out"=w323:errorcluster, "EncoderDevRef"=w324:T9)  [unwired: 5 in, 2 out]
              n143 = call <vilib>:"WPI_EncoderGet.vi"("error in (no error)"=w323, "EncoderDevRef"=w324) -> ("Distance"=w322:dbl)  [unwired: 4 in, 5 out]
              n144 = call <vilib>:"WPI_RobotDriveRefNum Registry Get.vi"("refnum name"="Left Right Motors") -> ("RobotDriveDevRef"=w349:T18)  [unwired: 9 in, 1 out]
              n145 = Equal?(x=w322, y=100.0) -> (x = y?=w320:bool)
              n146 = case shown="True" w320 {
                tunnel: w349 -> [w379 w383]
                tunnel: [w379 w380] -> w348
                frame False {
                }
                frame True {
                  n147 = call-poly <vilib>:"WPI_RobotDriveArcadeDrive.vi"("Y axis value"=0.05, "X axis value"=0.0, "RobotDriveDevRef"=w383) -> ("RobotDriveDevRef"=w380:T18)  [unwired: 6 in, 2 out]
                }
              }
              n148 = call <vilib>:"WPI_DigitalInputOpen.vi"("DIO Channel"=w318) -> ("DigitalInputDevRef"=w315:T4)  [unwired: 1 in, 9 out]
              n149 = call <vilib>:"WPI_DigitalInputOpen.vi"("DIO Channel"=w319) -> ("DigitalInputDevRef"=w316:T4)  [unwired: 1 in, 9 out]
              n150 = call-poly <vilib>:"WPI_CounterToDigitalSource.vi"("DigitalInputDevRef"=w315) -> ("Digital Source"=w314:T5)  [unwired: 6 out]
              n151 = call-poly <vilib>:"WPI_CounterToDigitalSource.vi"("DigitalInputDevRef"=w316) -> ("Digital Source"=w317:T5)  [unwired: 6 out]
              n152 = call <vilib>:"WPI_EncoderOpen.vi"("DistancePerCount"=18.84955592153876, "BSource"=w317, "ASource"=w314) -> ("error out"=w311:errorcluster, "EncoderDevRef"=w312:T9)  [unwired: 5 in, 2 out]
              n153 = call <vilib>:"WPI_EncoderGet.vi"("error in (no error)"=w311, "EncoderDevRef"=w312) -> ("Distance"=w310:dbl)  [unwired: 4 in, 5 out]
              n154 = call <vilib>:"WPI_RobotDriveDelayAndUpdateSafety.vi"("Delay (s)"=0.07, "RobotDriveDevRef"=w348) -> ("RobotDriveDevRef 2"=w344:T18)  [unwired: 8 in, 1 out]
              n155 = Equal?(x=w310, y=100.0) -> (x = y?=w308:bool)
              n156 = case shown="True" w308 {
                tunnel: w344 -> [w374 w378]
                tunnel: [w374 w375] -> w346
                frame False {
                }
                frame True {
                  n157 = call-poly <vilib>:"WPI_RobotDriveArcadeDrive.vi"("Y axis value"=0.15, "X axis value"=0.0, "RobotDriveDevRef"=w378) -> ("RobotDriveDevRef"=w375:T18)  [unwired: 6 in, 2 out]
                }
              }
              n158 = call <vilib>:"WPI_DigitalInputOpen.vi"("DIO Channel"=w306) -> ("DigitalInputDevRef"=w303:T4)  [unwired: 1 in, 9 out]
              n159 = call <vilib>:"WPI_DigitalInputOpen.vi"("DIO Channel"=w307) -> ("DigitalInputDevRef"=w304:T4)  [unwired: 1 in, 9 out]
              n160 = call-poly <vilib>:"WPI_CounterToDigitalSource.vi"("DigitalInputDevRef"=w303) -> ("Digital Source"=w302:T5)  [unwired: 6 out]
              n161 = call-poly <vilib>:"WPI_CounterToDigitalSource.vi"("DigitalInputDevRef"=w304) -> ("Digital Source"=w305:T5)  [unwired: 6 out]
              n162 = call <vilib>:"WPI_EncoderOpen.vi"("DistancePerCount"=18.84955592153876, "BSource"=w305, "ASource"=w302) -> ("error out"=w299:errorcluster, "EncoderDevRef"=w300:T9)  [unwired: 5 in, 2 out]
              n163 = call <vilib>:"WPI_EncoderGet.vi"("error in (no error)"=w299, "EncoderDevRef"=w300) -> ("Distance"=w298:dbl)  [unwired: 4 in, 5 out]
              n164 = call <vilib>:"WPI_RobotDriveDelayAndUpdateSafety.vi"("Delay (s)"=0.1, "RobotDriveDevRef"=w346) -> ("RobotDriveDevRef 2"=w341:T18)  [unwired: 8 in, 1 out]
              n165 = Equal?(x=w298, y=100.0) -> (x = y?=w296:bool)
              n166 = case shown="True" w296 {
                tunnel: w341 -> [w369 w373]
                tunnel: [w369 w370] -> w343
                frame False {
                }
                frame True {
                  n167 = call-poly <vilib>:"WPI_RobotDriveArcadeDrive.vi"("Y axis value"=0.3, "X axis value"=0.0, "RobotDriveDevRef"=w373) -> ("RobotDriveDevRef"=w370:T18)  [unwired: 6 in, 2 out]
                }
              }
              n168 = call <vilib>:"WPI_DigitalInputOpen.vi"("DIO Channel"=w294) -> ("DigitalInputDevRef"=w291:T4)  [unwired: 1 in, 9 out]
              n169 = call <vilib>:"WPI_DigitalInputOpen.vi"("DIO Channel"=w295) -> ("DigitalInputDevRef"=w292:T4)  [unwired: 1 in, 9 out]
              n170 = call-poly <vilib>:"WPI_CounterToDigitalSource.vi"("DigitalInputDevRef"=w291) -> ("Digital Source"=w290:T5)  [unwired: 6 out]
              n171 = call-poly <vilib>:"WPI_CounterToDigitalSource.vi"("DigitalInputDevRef"=w292) -> ("Digital Source"=w293:T5)  [unwired: 6 out]
              n172 = call <vilib>:"WPI_EncoderOpen.vi"("DistancePerCount"=18.84955592153876, "BSource"=w293, "ASource"=w290) -> ("error out"=w287:errorcluster, "EncoderDevRef"=w288:T9)  [unwired: 5 in, 2 out]
              n173 = call <vilib>:"WPI_EncoderGet.vi"("error in (no error)"=w287, "EncoderDevRef"=w288) -> ("Distance"=w286:dbl)  [unwired: 4 in, 5 out]
              n174 = call <vilib>:"WPI_RobotDriveDelayAndUpdateSafety.vi"("Delay (s)"=0.1, "RobotDriveDevRef"=w343) -> ("RobotDriveDevRef 2"=w339:T18)  [unwired: 8 in, 1 out]
              n175 = Equal?(x=w286, y=100.0) -> (x = y?=w284:bool)
              n176 = case shown="True" w284 {
                tunnel: w339 -> [w364 w368]
                tunnel: [w364 w365] -> w340
                frame False {
                }
                frame True {
                  n177 = call-poly <vilib>:"WPI_RobotDriveArcadeDrive.vi"("Y axis value"=0.5, "X axis value"=0.0, "RobotDriveDevRef"=w368) -> ("RobotDriveDevRef"=w365:T18)  [unwired: 6 in, 2 out]
                }
              }
              n178 = call <vilib>:"WPI_DigitalInputOpen.vi"("DIO Channel"=w282) -> ("DigitalInputDevRef"=w279:T4)  [unwired: 1 in, 9 out]
              n179 = call <vilib>:"WPI_DigitalInputOpen.vi"("DIO Channel"=w283) -> ("DigitalInputDevRef"=w280:T4)  [unwired: 1 in, 9 out]
              n180 = call-poly <vilib>:"WPI_CounterToDigitalSource.vi"("DigitalInputDevRef"=w279) -> ("Digital Source"=w278:T5)  [unwired: 6 out]
              n181 = call-poly <vilib>:"WPI_CounterToDigitalSource.vi"("DigitalInputDevRef"=w280) -> ("Digital Source"=w281:T5)  [unwired: 6 out]
              n182 = call <vilib>:"WPI_EncoderOpen.vi"("DistancePerCount"=18.84955592153876, "BSource"=w281, "ASource"=w278) -> ("error out"=w275:errorcluster, "EncoderDevRef"=w276:T9)  [unwired: 5 in, 2 out]
              n183 = call <vilib>:"WPI_EncoderGet.vi"("error in (no error)"=w275, "EncoderDevRef"=w276) -> ("Distance"=w274:dbl)  [unwired: 4 in, 5 out]
              n184 = call <vilib>:"WPI_RobotDriveDelayAndUpdateSafety.vi"("Delay (s)"=0.1, "RobotDriveDevRef"=w340) -> ("RobotDriveDevRef 2"=w335:T18)  [unwired: 8 in, 1 out]
              n185 = Equal?(x=w274, y=100.0) -> (x = y?=w261:bool)
              n186 = case shown="True" w261 {
                tunnel: w335 -> [w359 w363]
                tunnel: [w359 w360] -> w336
                frame False {
                }
                frame True {
                  n187 = call-poly <vilib>:"WPI_RobotDriveArcadeDrive.vi"("Y axis value"=0.7, "X axis value"=0.0, "RobotDriveDevRef"=w363) -> ("RobotDriveDevRef"=w360:T18)  [unwired: 6 in, 2 out]
                }
              }
              n188 = call <vilib>:"WPI_DigitalInputOpen.vi"("DIO Channel"=w271) -> ("DigitalInputDevRef"=w268:T4)  [unwired: 1 in, 9 out]
              n189 = call <vilib>:"WPI_DigitalInputOpen.vi"("DIO Channel"=w272) -> ("DigitalInputDevRef"=w269:T4)  [unwired: 1 in, 9 out]
              n190 = call-poly <vilib>:"WPI_CounterToDigitalSource.vi"("DigitalInputDevRef"=w268) -> ("Digital Source"=w267:T5)  [unwired: 6 out]
              n191 = call-poly <vilib>:"WPI_CounterToDigitalSource.vi"("DigitalInputDevRef"=w269) -> ("Digital Source"=w270:T5)  [unwired: 6 out]
              n192 = call <vilib>:"WPI_EncoderOpen.vi"("DistancePerCount"=18.84955592153876, "BSource"=w270, "ASource"=w267) -> ("error out"=w264:errorcluster, "EncoderDevRef"=w265:T9)  [unwired: 5 in, 2 out]
              n193 = call <vilib>:"WPI_EncoderGet.vi"("error in (no error)"=w264, "EncoderDevRef"=w265) -> ("Distance"=w263:dbl)  [unwired: 4 in, 5 out]
              n194 = call <vilib>:"WPI_RobotDriveDelayAndUpdateSafety.vi"("Delay (s)"=0.1, "RobotDriveDevRef"=w336) -> ("RobotDriveDevRef 2"=w332:T18)  [unwired: 8 in, 1 out]
              n195 = Equal?(x=w263, y=100.0) -> (x = y?=w260:bool)
              n196 = case shown="True" w260 {
                tunnel: w332 -> [w354 w358]
                tunnel: [w354 w355] -> w333
                frame False {
                }
                frame True {
                  n197 = call-poly <vilib>:"WPI_RobotDriveArcadeDrive.vi"("Y axis value"=0.9, "X axis value"=0.0, "RobotDriveDevRef"=w358) -> ("RobotDriveDevRef"=w355:T18)  [unwired: 6 in, 2 out]
                }
              }
              n198 = call <vilib>:"WPI_DigitalInputOpen.vi"("DIO Channel"=w258) -> ("DigitalInputDevRef"=w255:T4)  [unwired: 1 in, 9 out]
              n199 = call <vilib>:"WPI_DigitalInputOpen.vi"("DIO Channel"=w259) -> ("DigitalInputDevRef"=w256:T4)  [unwired: 1 in, 9 out]
              n200 = call-poly <vilib>:"WPI_CounterToDigitalSource.vi"("DigitalInputDevRef"=w255) -> ("Digital Source"=w254:T5)  [unwired: 6 out]
              n201 = call-poly <vilib>:"WPI_CounterToDigitalSource.vi"("DigitalInputDevRef"=w256) -> ("Digital Source"=w257:T5)  [unwired: 6 out]
              n202 = call <vilib>:"WPI_EncoderOpen.vi"("DistancePerCount"=18.84955592153876, "BSource"=w257, "ASource"=w254) -> ("error out"=w251:errorcluster, "EncoderDevRef"=w252:T9)  [unwired: 5 in, 2 out]
              n203 = call <vilib>:"WPI_EncoderGet.vi"("error in (no error)"=w251, "EncoderDevRef"=w252) -> ("Distance"=w250:dbl)  [unwired: 4 in, 5 out]
              n204 = call <vilib>:"WPI_RobotDriveDelayAndUpdateSafety.vi"("Delay (s)"=0.1, "RobotDriveDevRef"=w333) -> ("RobotDriveDevRef 2"=w331:T18)  [unwired: 8 in, 1 out]
              n205 = Equal?(x=w250, y=100.0) -> (x = y?=w248:bool)
              n206 = case shown="True" w248 {
                tunnel: w331 -> [_ w353]
                frame False {
                }
                frame True {
                  n207 = call-poly <vilib>:"WPI_RobotDriveArcadeDrive.vi"("Y axis value"=0.5, "X axis value"=0.0, "RobotDriveDevRef"=w353) -> ()  [unwired: 6 in, 3 out]
                }
              }
            }
          }
        }
      }
    }
    frame Enabled {
    }
  }
